vi "Write Controls of Panel to INI.vi"(5 "float number format (optional)":string, 6 "Rep":string="^[!@#$%^&*-_+]", 8 "error in (no error)":errorcluster, 10 "VI Ref (calling VI)":refnum<vi>, 11 "refnum":T1) -> (0 "error out":errorcluster, 3 "refnum out":T1)   [LabVIEW 2017]
doc: "Writes the values of the front panel controls of VI Ref to a LabVIEW configuration (INI) file as key-value pairs. Use it together with Read Controls of Panel from INI.vi."
uses:
  <vilib>/Utility/config.llb/Config Data RefNum.ctl
  _OpenG Variant Configuration File/OpenG Variant Configuration File.lvlib
  <vilib>/Utility/config.llb/NI_LVConfig.lvlib
panel:
  # "Write Panel to INI.vi\n\nWrites all Front Panel data to INI file.\n\nPlease visit http://www.OpenG.org to learn about the\nOpen Source LabVIEW software movement.\n\nNOTICE -- YOU MUST LEAVE THIS NOTICE IN PLACE.  PER THE TERMS OF THE LICENSE BELOW, YOU MAY SUBLICENSE THIS SOFTWARE \nIN ANY WAY THAT DOES NOT CONFLICT WITH THIS LICENSE.\n\n### BSD License (http://www.opensource.org/licenses/bsd-license.php) Begin ###\n \nCopyright (c) 2002, Jean-Pierre Drolet <drolet_jp@hotmail.com>\n\nAll rights reserved.\n\nRedistribution and use in source and binary forms, with or without modification, are permitted provided that the following conditions are met:\n\n    * Redistributions of source code must retain the above copyright notice, this list of conditions and the following disclaimer.\n    * Redistributions in binary form must reproduce the above copyright notice, this list of conditions and the following disclaimer in the \n       documentation and/or other materials provided with the distribution.\n    * Neither the name of SciWare, James Kring, Inc., nor the names of its contributors may be used to endorse or promote products derived \n       from this software without specific prior written permission.\n\nTHIS SOFTWARE IS PROVIDED BY THE COPYRIGHT HOLDERS AND CONTRIBUTORS \"AS IS\" AND ANY EXPRESS OR IMPLIED WARRANTIES, \nINCLUDING, BUT NOT LIMITED TO, THE IMPLIED WARRANTIES OF MERCHANTABILITY AND FITNESS FOR A PARTICULAR PURPOSE ARE \nDISCLAIMED. IN NO EVENT SHALL THE COPYRIGHT OWNER OR CONTRIBUTORS BE LIABLE FOR ANY DIRECT, INDIRECT, INCIDENTAL,\n SPECIAL, EXEMPLARY, OR CONSEQUENTIAL DAMAGES (INCLUDING, BUT NOT LIMITED TO, PROCUREMENT OF SUBSTITUTE GOODS OR \nSERVICES; LOSS OF USE, DATA, OR PROFITS; OR BUSINESS INTERRUPTION) HOWEVER CAUSED AND ON ANY THEORY OF LIABILITY, \nWHETHER IN CONTRACT, STRICT LIABILITY, OR TORT (INCLUDING NEGLIGENCE OR OTHERWISE) ARISING IN ANY WAY OUT OF THE USE \nOF THIS SOFTWARE, EVEN IF ADVISED OF THE POSSIBILITY OF SUCH DAMAGE.\n\n### BSD License End ###"
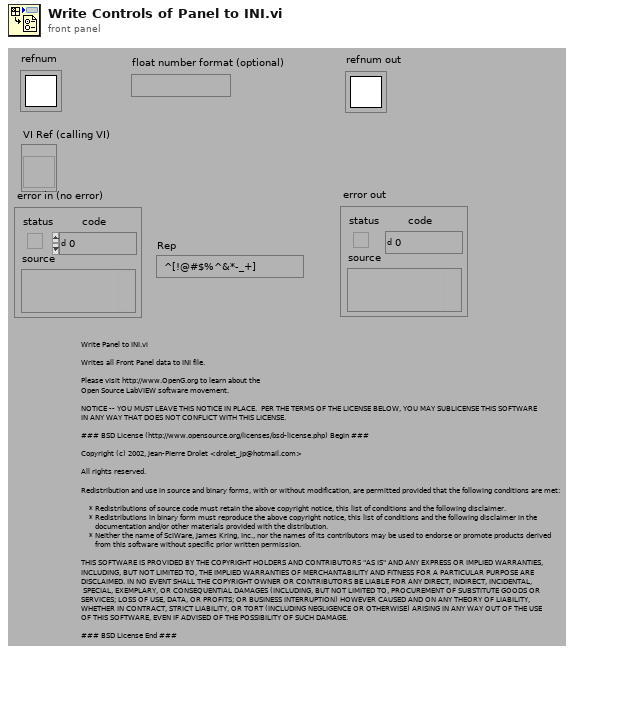
[diagram p1: front panel]
types:
  T1 = typedef "NI_LVConfig.lvlib/Config Data RefNum.ctl" = refnum<k1>
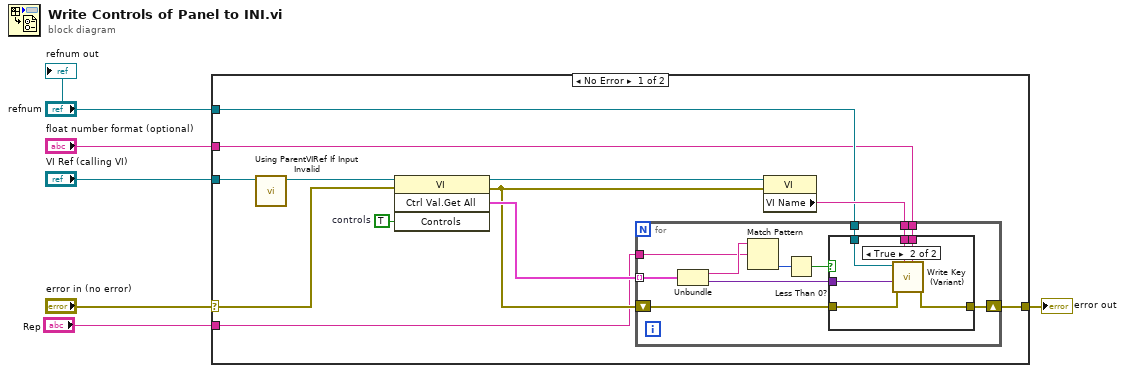
[diagram p0: block diagram]
diagram:
  n1 = case shown="No Error" "error in (no error)" {
    selector: "error in (no error)" -> [w11 w37]
    tunnel: "refnum" -> [w13 _]
    tunnel: [w12 w37] -> w5
    tunnel: "VI Ref (calling VI)" -> [w8 _]
    tunnel: "float number format (optional)" -> [w10 _]
    tunnel: "Rep" -> [w9 _]
    frame No Error {
      w18 = TRUE  # controls
      n2 = call "Using ParentVIRef If Input Invalid.vi"("VI Ref (calling VI)"=w8) -> ("VI Ref"=w7:refnum<vi>)  [unwired: 5 in, 1 out]
      n3 = invoke class="VI" method="Ctrl Val.Get All"(reference=w7, error in=w11, "Controls"=w18) -> (reference out=w17:refnum<vi>, error out=w15:errorcluster, "Get All Control Values Variant"=w16:cluster{"Name":string, "Variant Data":variant}[])  [unwired: 1 in, 1 out]
      n4 = property class="VI"(reference=w17, error in=w15) -> ("VI Name"=w14:string)  [unwired: 2 out]
      n5 = for {
        tunnel: w16 -> [w29] mode=indexing
        tunnel: w14 -> [w28]
        tunnel: w13 -> [w27]
        shift-right: [w26] -> w12
        shift-left: w15 -> [w23]
        tunnel: w10 -> [w25]
        tunnel: w9 -> [w19]
        n6 = Unbundle(w29) -> ("Name"=w22:string, "Variant Data"=w24:variant)
        n7 = Match Pattern(string=w22, regular expression=w19) -> (offset past match=w21:i32)  [unwired: 1 in, 3 out]
        n8 = Less Than 0?(x=w21) -> (x < 0?=w20:bool)
        n9 = case shown="True" w20 {
          tunnel: w28 -> [_ w36]
          tunnel: w27 -> [_ w35]
          tunnel: [w30 w34] -> w26
          tunnel: w25 -> [_ w33]
          tunnel: w24 -> [_ w32]
          tunnel: w23 -> [w30 w31]
          frame False {
          }
          frame True {
            n10 = call "Write Key (Variant).vi"("float number format"=w33, "section"=w36, "error in (no error)"=w31, "key-value"=w32, "refnum"=w35) -> ("error out"=w34:errorcluster)  [unwired: 5 in, 1 out]
          }
        }
      }
    }
    frame Error {
    }
  }
  "error out" <- w5
  "refnum out" <- "refnum"
